vi "y1y2 (子VI)备份3.vi"(0 "Image Pixels (U8)输入":u8[][](array[numeric])) -> (5 "left":cluster{i32, i32}[](graph), 6 "out left point":cluster{i32, i32}[](array[cluster]), 7 "right":cluster{i32, i32}[](graph), 8 "out right point 2":cluster{i32, i32}[](array[cluster]))   [LabVIEW 2014]
panel:
  out "x2max":cluster{i32, i32}
  out "x2min":cluster{i32, i32}
  out "x1min":cluster{i32, i32}
  out "x1max":cluster{i32, i32}
  # "x"
  # "1"
  # "2"
  # "y"
  # "x"
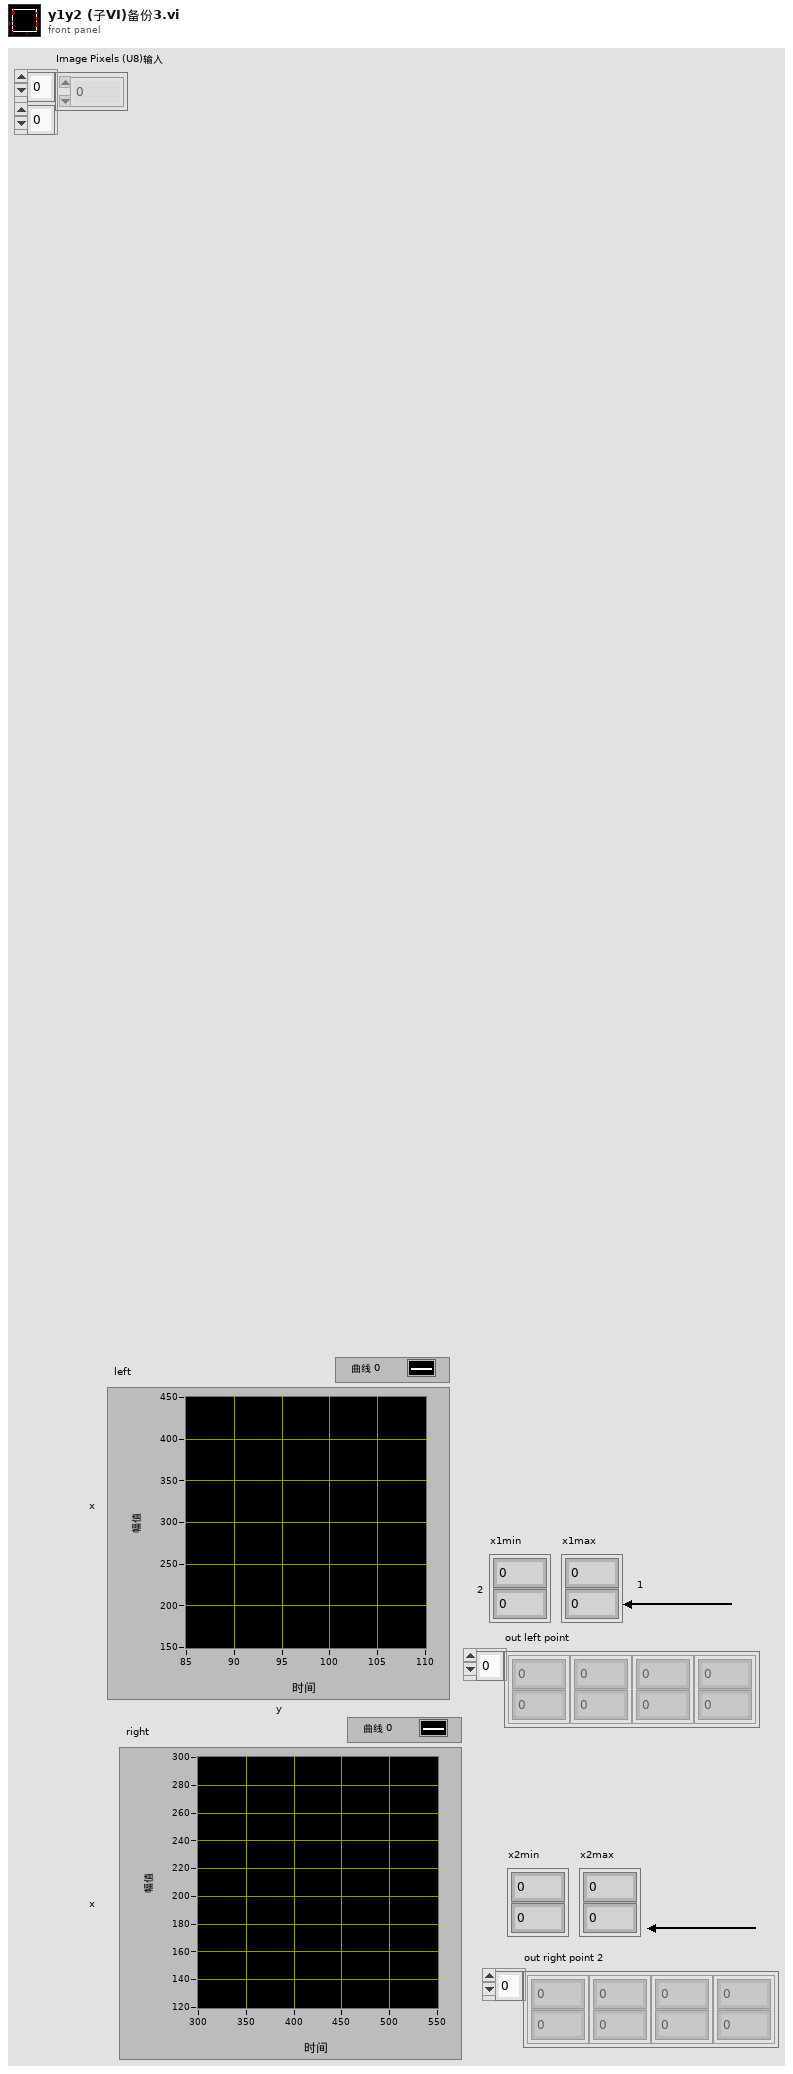
[diagram p1: front panel]
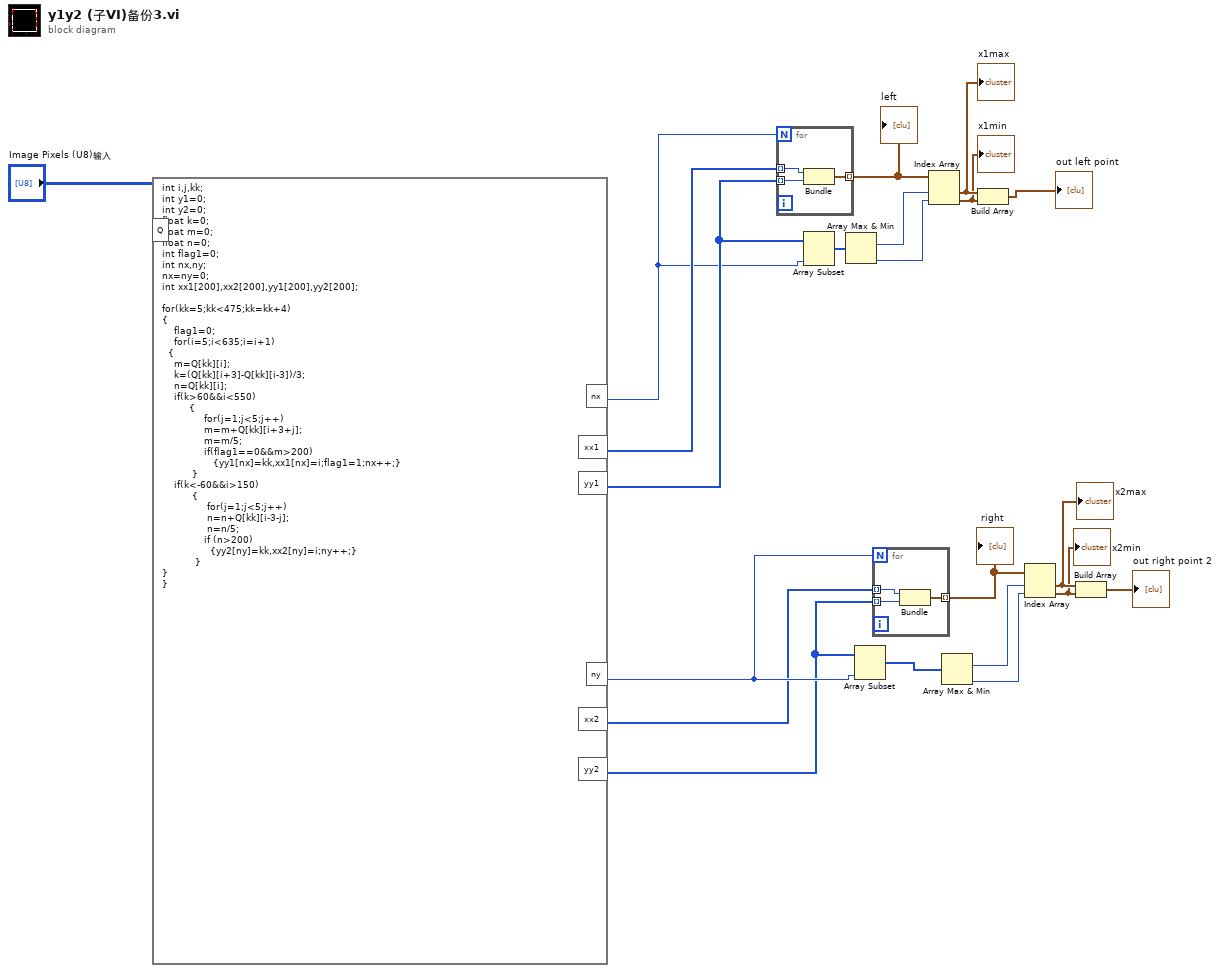
[diagram p0: block diagram]
diagram:
  n1 = formula code="int i,j,kk;\nint y1=0;\nint y2=0;\nfloat k=0;\nfloat m=0;\nfloat n=0;\nint flag1=0;\nint nx,ny;\nnx=ny=0;\nint xx1[200],xx2[200],yy1[200],yy2[200];\n\nfor(kk=5;kk<475;kk=kk+4)\n{\n    flag1=0;\n    for(i=5;i<635;i=i+1)\n  {\n    m=Q[kk][i];\n    k=(Q[kk][i+3]-Q[kk][i-3])/3;\n    n=Q[kk][i];\n    if(k>60&&i<550)\n         {   \n              for(j=1;j<5;j++)\n              m=m+Q[kk][i+3+j];\n              m=m/5;\n              if(flag1==0&&m>200)\n                 {yy1[nx]=kk,xx1[nx]=i;flag1=1;nx++;}\n          }\n    if(k<-60&&i>150)\n          {                   \n               for(j=1;j<5;j++)\n               n=n+Q[kk][i-3-j];\n               n=n/5;\n              if (n>200)\n                {yy2[ny]=kk,xx2[ny]=i;ny++;}\n           }\n}\n}"("Q"="Image Pixels (U8)输入") -> ("xx1"=w17:i32[], "yy1"=w18:i32[], "nx"=w16:i32, "xx2"=w10:i32[], "yy2"=w11:i32[], "ny"=w12:i32)
  n2 = for {
    N: w16 -> [_]
    tunnel: w17 -> [w24] mode=indexing
    tunnel: w18 -> [w23] mode=indexing
    tunnel: [w22] -> w21 mode=indexing
    n3 = Bundle(w24, w23) -> (w22:cluster{i32, i32})  [unwired: 1 in]
  }
  "left" <- w21
  n4 = Array Subset(array=w18, length=w16) -> (w3:i32[])  [unwired: 1 in]
  n5 = Array Max & Min(array=w3) -> (max index (indices)=w20:i32, min index (indices)=w19:i32)  [unwired: 2 out]
  n6 = Array Subset(array=w11, length=w12) -> (w1:i32[])  [unwired: 1 in]
  n7 = for {
    N: w12 -> [_]
    tunnel: w10 -> [w27] mode=indexing
    tunnel: w11 -> [w26] mode=indexing
    tunnel: [w25] -> w13 mode=indexing
    n8 = Bundle(w27, w26) -> (w25:cluster{i32, i32})  [unwired: 1 in]
  }
  "right" <- w13
  n9 = Index Array(array=w21, index #1=w20, index #2=w19) -> (element #1=w8:cluster{i32, i32}, element #2=w7:cluster{i32, i32})
  "x1max" <- w8
  "x1min" <- w7
  n10 = Array Max & Min(array=w1) -> (max index (indices)=w14:i32, min index (indices)=w15:i32)  [unwired: 2 out]
  n11 = Build Array(w8, w7) -> (→"out left point":cluster{i32, i32}[])
  n12 = Index Array(array=w13, index #1=w14, index #2=w15) -> (element #1=w5:cluster{i32, i32}, element #2=w4:cluster{i32, i32})
  "x2max" <- w5
  "x2min" <- w4
  n13 = Build Array(w5, w4) -> (→"out right point 2":cluster{i32, i32}[])
